vi "Thread@SubThreadScript__Parameter.vi"(1 "ParamterIn":string) -> (0 "ParamterOut":string)   [LabVIEW 2020]
uses:
  MainFrame/Global.vi
panel:
  in  "Section":string(combo)
  in  "Script":string(combo)
  in  "SubName":string(combo)
  in  "Confirm":bool
  # "Thread@SubThreadScript $SubName,$Script(,$Section)"
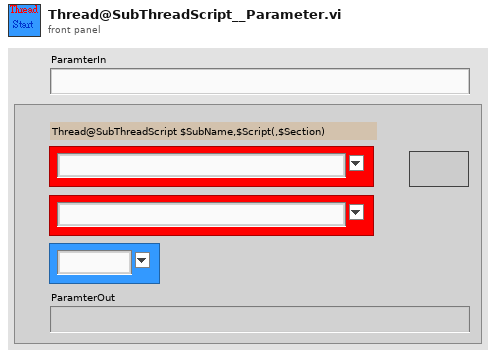
[diagram p1: front panel]
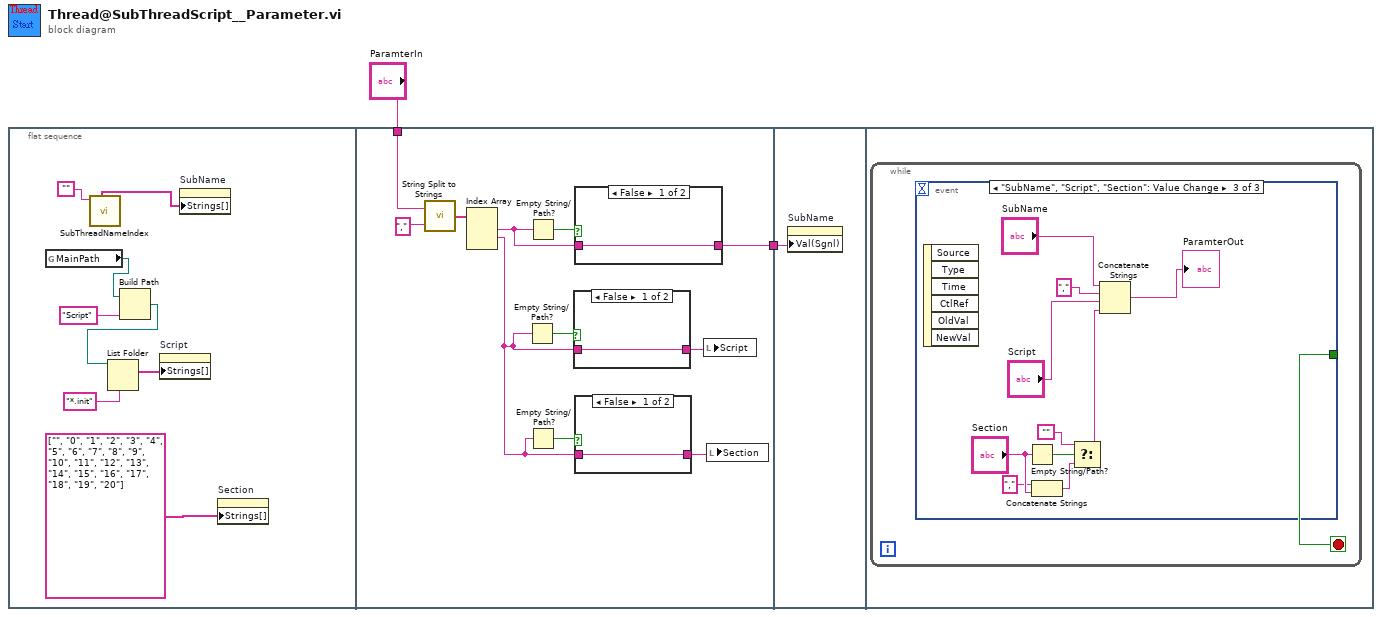
[diagram p0: block diagram]
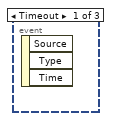
[diagram p5: hidden frame]
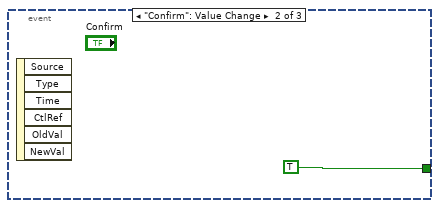
[diagram p6: hidden frame]
diagram:
  n1 = flat-sequence {
    tunnel: "ParamterIn" -> [w19]
    tunnel: [w16] -> w1
    tunnel: w1 -> [w25]
    frame #0 {
      n2 = global read "Global.vi" "MainPath"() -> (w10:path)
      n3 = call "SubThreadNameIndex.vi"("SubThreadName"="") -> ("SubThread Name"=w6:string[])  [unwired: 7 in, 3 out]
      n4 = Build Path(base path=w10, name or relative path="Script") -> (appended path=w8:path)
      n5 = List Folder(path=w8, pattern="*.init") -> (filenames=w5:string[])  [unwired: 2 in, 3 out]
      n6 = property on="Script" class="CmbBox"("Strings[]"=w5) -> ()  [unwired: 2 in, 2 out]
      n7 = property on="SubName" class="CmbBox"("Strings[]"=w6) -> ()  [unwired: 2 in, 2 out]
      n8 = property on="Section" class="CmbBox"("Strings[]"=string[] ["", "0", "1", "2", "3", "4", "5", "6", "7", "8", "9", "10", "11", "12", "13", "14", "15", "16", "17", "18", "19", "20"] ("Strings []")) -> ()  [unwired: 2 in, 2 out]
    }
    frame #1 {
      n9 = call "String Split to Strings.vi"("search string/char (-)"=",", "String"=w19) -> ("Array"=w21:string[])
      n10 = Index Array(array=w21) -> (element #1=w17:string, element #2=w12:string)  [unwired: 3 in, 1 out]
      n11 = Empty String/Path?(string/path=w12) -> (empty?=w15:bool)
      n12 = Empty String/Path?(string/path=w17) -> (empty?=w18:bool)
      n13 = Empty String/Path?(string/path=w12) -> (empty?=w13:bool)
      n14 = case shown="False" w15 {
        tunnel: w12 -> [w23 _]
        tunnel: [w23 _] -> w14
        frame False {
        }
        frame True {
        }
      }
      n15 = case shown="False" w18 {
        tunnel: w17 -> [w24 _]
        tunnel: [w24 _] -> w16
        frame False {
        }
        frame True {
        }
      }
      n16 = case shown="False" w13 {
        tunnel: w12 -> [w22 _]
        tunnel: [w22 _] -> w11
        frame False {
        }
        frame True {
        }
      }
      n17 = local write "Script"(w14) -> ()
      n18 = local write "Section"(w11) -> ()
    }
    frame #2 {
      n19 = property on="SubName" class="CmbBox"("Val(Sgnl)"=w25) -> ()  [unwired: 2 in, 2 out]
    }
    frame #3 {
      n20 = while {
        stop <- w26 stop-if-true
        n21 = event shown="[2] \"SubName\", \"Script\", \"Section\": Value Change" {
          selector: _ -> [_ _ _]
          dyn-events: _ -> [_ _ _]
          timeout: _ -> [_ _ _]
          tunnel: [_ TRUE _] -> w26
          event Timeout {
            n22 = event-data() -> ()  [unwired: 1 in, 3 out]
          }
          event "Confirm": Value Change {
            n23 = event-data() -> ()  [unwired: 1 in, 6 out]
          }
          event "SubName", "Script", "Section": Value Change {
            n24 = event-data() -> ()  [unwired: 1 in, 6 out]
            n25 = Empty String/Path?(string/path="Section") -> (empty?=w33:bool)
            n26 = Concatenate Strings("," ("string"), "Section") -> (w31:string)
            n27 = Select(t="", s=w33, f=w31) -> (s? t:f=w28:string)
            n28 = Concatenate Strings("SubName", "," ("string"), "Script", w28) -> (→"ParamterOut":string)
          }
        }
      }
    }
  }
